vi "PH_AxisGUI_BaseClass.ProcEvents.vi"(0 "i ref in":refnum<vi>, 5 "error in":errorcluster) -> (14 "i ref out":refnum<vi>, 19 "error out":errorcluster)   [LabVIEW 2014, in "PH_AxisGUI_BaseClass.lvlib"]
doc: "This method is used to define the events the object will listen to. Add your own events here."
uses:
  PH_AxisGUI_BaseClass.lvlib
  PH_Stepmotor_BaseClass/PH_Stepmotor_BaseClass.Axis DIM Tags.ctl
  PH_Common/DIM/PH_DIM.Event Declarer.ctl
  CS_Core/BaseProcess/BaseProcess.lvlib
  PH_Stepmotor_BaseClass/PH_Stepmotor_BaseClass.lvlib
  PH_Common/PH_Common.lvlib
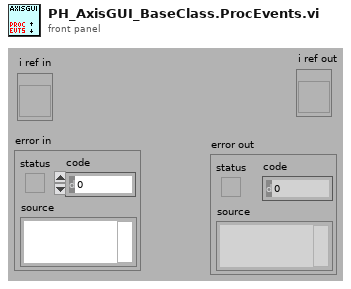
[diagram p1: front panel]
types:
  T1 = typedef "PH_Common.lvlib/PH_DIM.Event Declarer.ctl" = cluster{"Service Name":string, "Selector":string}
  T2 = typedef "PH_Stepmotor_BaseClass.lvlib/PH_Stepmotor_BaseClass.Axis DIM Tags.ctl" = enum16{"no Info", "Information", "Settings"}
  T3 = typedef "PH_AxisGUI_BaseClass.lvlib/PH_AxisGUI_BaseClass.i attribute.ctl" = cluster{"Axes":T4[]}
  T4 = typedef "PH_AxisGUI_BaseClass.lvlib/PH_AxisGUI_BaseClass.Axis Attributes.ctl" = cluster{"Axis GUI Refs":T5, "Address":T6, "Name":string, "Label \"Back\"":string, "Labell \"Forth\"":string, "Moving?":bool}
  T5 = typedef "PH_AxisGUI_BaseClass.lvlib/PH_AxisGUI_BaseClass.Axis GUI Refs.ctl" = cluster{"Back":refnum<vi>, "Forth":refnum<vi>, "Status":refnum<vi>, "Target":refnum<vi>, "Address":refnum<vi>, "Status Bar":refnum<vi>, "Settings":refnum<vi>, "Activity":refnum<vi>, "Clear Error":refnum<vi>}
  T6 = typedef "PH_Stepmotor_BaseClass.lvlib/PH_Stepmotor_BaseClass.Axis Address.ctl" = cluster{"Instance":string, "Motor Nr":i32}
  T7 = typedef "BaseProcess.lvlib/BaseProcess.event definition.ctl" = cluster{"CAEEvtDef":T8, "Data Descriptor":T9}
  T8 = typedef "CAEObj.lvlib/CAEObj.event definition.ctl" = cluster{"URL":string, "enable":bool, "ignoreResID":bool}
  T9 = typedef "BaseProcess.lvlib/BaseProcess.descriptor string definition.ctl" = string
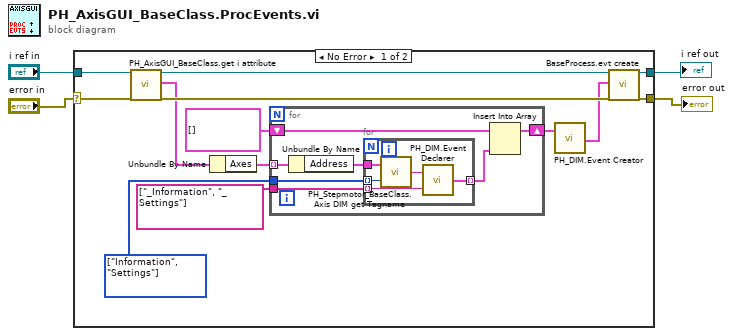
[diagram p0: block diagram]
diagram:
  n1 = case shown="No Error" "error in" {
    selector: "error in" -> [w15 w30]
    tunnel: "i ref in" -> [w13 w31]
    tunnel: [w17 w31] -> w3
    tunnel: [w16 w30] -> w2
    frame No Error {
      w10 = T2[] [enum."Information", enum."Settings"] items=["no Info", "Information", "Settings"]
      n2 = call "PH_AxisGUI_BaseClass.get i attribute.vi"("i ref in"=w13, "error in (no error)"=w15) -> ("i ref out"=w12:refnum<vi>, "i attribute"=w8:T3, "error out"=w14:errorcluster)  [unwired: 15 in]
      n3 = Unbundle By Name(w8) -> ("Axes"=w6:T4[])
      n4 = for {
        tunnel: w10 -> [w23]
        tunnel: string[] ["_Information", "_Settings"] -> [w22]
        tunnel: w6 -> [w21] mode=indexing
        shift-right: [w24] -> w11
        shift-left: T1[] [] -> [w18]
        n5 = Unbundle By Name(w21) -> ("Address"=w20:T6)
        n6 = for {
          tunnel: [w29] -> w19 mode=indexing
          tunnel: w22 -> [w28] mode=indexing
          tunnel: w20 -> [w26]
          tunnel: w23 -> [w25] mode=indexing
          n7 = call "PH_Stepmotor_BaseClass.Axis DIM get Tagname.vi"("Tag"=w25, "Instancename"=w26) -> ("Axis Tagname"=w27:string)
          n8 = call "PH_DIM.Event Declarer.vi"("Selector"=w28, "Service Name"=w27) -> ("declared DIM Event"=w29:T1)
        }
        n9 = Insert Into Array(array=w18, new element=w19) -> (w24:T1[])  [unwired: 1 in]
      }
      n10 = call "PH_DIM.Event Creator.vi"("Trendmessage Services"=w11) -> ("DIM Service Events"=w7:T7[])  [unwired: 18 in]
      n11 = call "BaseProcess.evt create.vi"("i ref in"=w12, "newEvents"=w7, "error in (no error)"=w14) -> ("i ref out"=w17:refnum<vi>, "error out"=w16:errorcluster)  [unwired: 13 in, 2 out]
    }
    frame Error {
    }
  }
  "i ref out" <- w3
  "error out" <- w2
